vi "Time calculator.vi"(9 "Previous Absolute Time":timestamp, 10 "Current Absolute Time":timestamp, 11 "Previous Relative Time":dbl) -> (2 "Absolute Time out":timestamp, 3 "Relative Time out":dbl)   [LabVIEW 2020]
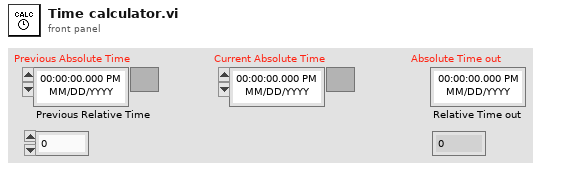
[diagram p1: front panel]
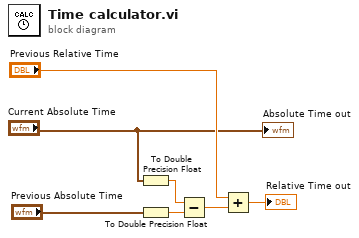
[diagram p0: block diagram]
diagram:
  n1 = To Double Precision Float(number="Current Absolute Time") -> (double precision float=w5:dbl)
  n2 = To Double Precision Float(number="Previous Absolute Time") -> (double precision float=w6:dbl)
  n3 = Subtract(x=w5, y=w6) -> (x-y=w4:dbl)
  n4 = Add(x="Previous Relative Time", y=w4) -> (x+y=→"Relative Time out":dbl)
  "Absolute Time out" <- "Current Absolute Time"
